vi "Host_continuousPathSamplingFPGA2.vi"() -> ()   [LabVIEW 2017]
uses:
  <vilib>/Utility/file.llb/Read From Spreadsheet File (I64).vi
  <vilib>/FPGAPlugInAG/cRIO-9082/niLvFpga_Open_cRIO-9082.vi
  <vilib>/rvi/interface/common/dynamic/niFpgaDynamicAddResources.vi
  <vilib>/FPGAPlugInAG/Dynamic/niLvFpga_Reset_Dynamic.vi
  <vilib>/Utility/error.llb/Error Cluster From Error Code.vi
  <vilib>/rvi/errors/niLvFpgaAdjustHostInterfaceError.vi
  <vilib>/rvi/interface/common/niFpgaWaitOnOcc.vi
  <vilib>/FPGAPlugInAG/Dynamic/niLvFpga_Run_Dynamic.vi
  <vilib>/Utility/file.llb/Write To Spreadsheet File (DBL).vi
  <vilib>/rvi/interface/nirviOpenFPGA/nirviOpenFPGA.xnode
  FPGA Bitfiles/simpletest_FPGATarget_coutinuousPathSa_wEIBsGw6M4w.lvbitx
  coutinuousPathSamplingFPGA4.vi
  <vilib>/rvi/interface/nirviMethod/nirviMethod.xnode
  <vilib>/rvi/interface/nirviReadWriteControl/nirviReadWriteControl.xnode
  <vilib>/rvi/interface/Simulation/niFpgaSimulationCallBeginRW.vi
  <vilib>/FPGAPlugInAG/Dynamic/niLvFpga_ConfigureFifo_Dynamic.vi
  <vilib>/rvi/errors/niLvFpgaMergeErrorWithErrorCode.vi
  NiFpgaLv.dll
  <vilib>/FPGAPlugInAG/Dynamic/niLvFpga_WriteFifo_Dynamic.vi
  <vilib>/FPGAPlugInAG/Dynamic/niLvFpga_StartFifo_Dynamic.vi
  <vilib>/FPGAPlugInAG/Dynamic/niLvFpga_ReadFifo_Dynamic.vi
panel:
  out "z output":dbl=5.1361083984375
  out "y output":dbl=3.794647216796875
  out "x output":dbl=-1.222381591796875
  out "deflection":dbl=-0.001068115234375
  out "z":dbl=-4.291839599609375
  out "y":dbl=3.9134521484375
  out "x":dbl=1.858306884765625
  out "Elements Remaining":u32=68432
  out "FINISH_SIGNAL":bool
  in  "stop":bool
  in  "scanning path file path":path=path "C:/Users/AnderssonLab/Desktop/yufan/sample locations/finalSamplingSeqRFD_continuous256MuPath50_8FOR14_1D2_1400_16ptg_1.txt"
  out "Empty Elements Remaining":u32
  out "Actual Depth":u32=24188
  in  "Threshold":T1={"x threshold"=0.02301025390625, "y threshold"=0.02301025390625, "z threshold"=0.5, "deflection threshold"=0.019989013671875}
  in  "ImageToSample":T2={"image size_x"=256, "image size_y"=256, "sample start_x"=0.0, "sample start_y"=0.0, "sample end_x"=6.0, "sample end_y"=6.0}
  in  "deflection control":T3={"SetPoint (V)"=0.0, "scanning I"=20.0, "scanning P"=0.01953125, "Initial I (V)"=0.0, "Upper Limit (V)"=9.900000095367432, "Lower Limit (V)"=-9.900000095367432}
  in  "z control":T4={"SetPoint (V)"=-1.0, "I"=100.0, "P"=0.0595703125, "Initial I (V)"=0.0, "Upper Limit (V)"=9.900000095367432, "Lower Limit (V)"=-9.900000095367432}
  in  "y control":T3={"SetPoint (V)"=0.0, "scanning I"=1850.0, "scanning P"=0.099609375, "Initial I (V)"=0.0, "Upper Limit (V)"=9.900000095367432, "Lower Limit (V)"=-9.900000095367432}
  in  "x control":T3={"SetPoint (V)"=0.0, "scanning I"=1850.0, "scanning P"=0.099609375, "Initial I (V)"=0.0, "Upper Limit (V)"=9.900000095367432, "Lower Limit (V)"=-9.900000095367432}
  in  "Clock (uSec)":T5={"XY Clock (uSec)"=20.0, "Z Clock (uSec)"=3.0, "Stage Clock (uSec)"=500.0, "muPathUpdate Clock (uSec)"=200.0, "Sampling Clock (uSec)"=4500.0, "pixel segment"=100}
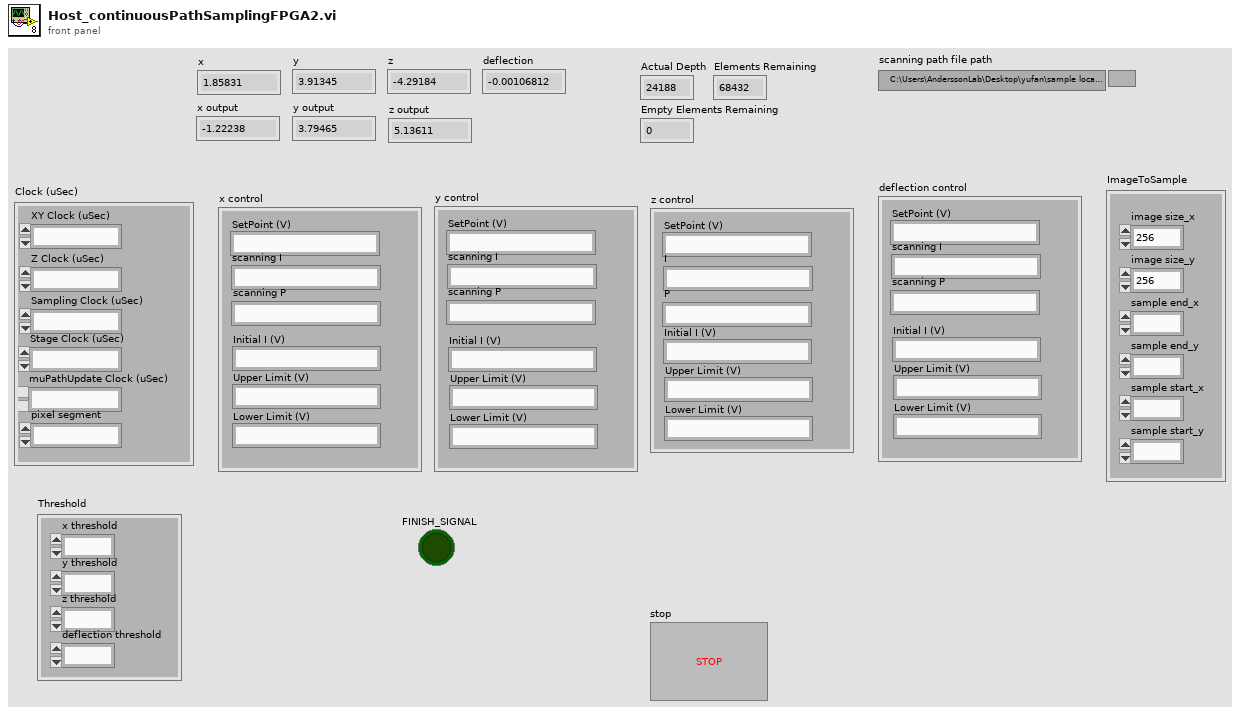
[diagram p1: front panel]
types:
  T1 = cluster{"x threshold":fxp<+/-,20,5>, "y threshold":fxp<+/-,20,5>, "z threshold":fxp<+/-,20,5>, "deflection threshold":fxp<+/-,20,5>}
  T2 = cluster{"image size_x":u16, "image size_y":u16, "sample start_x":fxp<+/-,26,5>, "sample start_y":fxp<+/-,26,5>, "sample end_x":fxp<+/-,26,5>, "sample end_y":fxp<+/-,26,5>}
  T3 = cluster{"SetPoint (V)":fxp<+/-,26,5>, "scanning I":fxp<+,21,13>, "scanning P":fxp<+,15,5>, "Initial I (V)":fxp<+/-,10,5>, "Upper Limit (V)":fxp<+/-,26,5>, "Lower Limit (V)":fxp<+/-,26,5>}
  T4 = cluster{"SetPoint (V)":fxp<+/-,26,5>, "I":fxp<+,21,13>, "P":fxp<+,15,5>, "Initial I (V)":fxp<+/-,10,5>, "Upper Limit (V)":fxp<+/-,26,5>, "Lower Limit (V)":fxp<+/-,26,5>}
  T5 = cluster{"XY Clock (uSec)":fxp<+,32,32>, "Z Clock (uSec)":fxp<+,32,32>, "Stage Clock (uSec)":fxp<+,32,32>, "muPathUpdate Clock (uSec)":fxp<+,32,32>, "Sampling Clock (uSec)":fxp<+,32,32>, "pixel segment":u32}
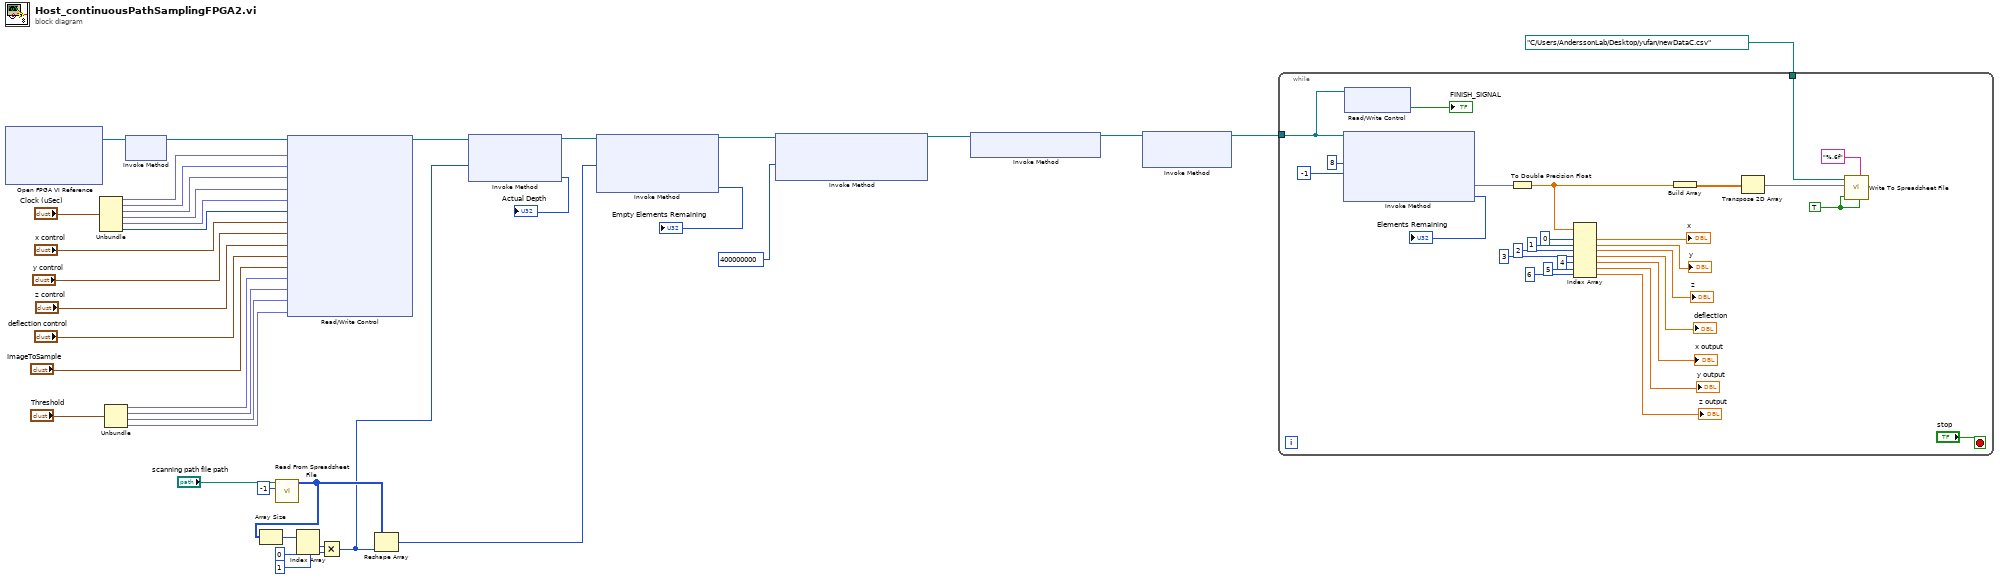
[diagram p0: block diagram]
diagram:
  n1 = xnode "Open FPGA VI Reference"() -> ("FPGA VI Reference Out"=w39:refnum<k20>)  [unwired: 2 in, 1 out]
  n2 = Unbundle("Clock (uSec)") -> ("XY Clock (uSec)"=w36:fxp<+,32,32>, "Z Clock (uSec)"=w35:fxp<+,32,32>, "Stage Clock (uSec)"=w34:fxp<+,32,32>, "muPathUpdate Clock (uSec)"=w33:fxp<+,32,32>, "Sampling Clock (uSec)"=w32:fxp<+,32,32>, "pixel segment"=w31:u32)
  n3 = Unbundle("Threshold") -> ("x threshold"=w24:fxp<+/-,20,5>, "y threshold"=w23:fxp<+/-,20,5>, "z threshold"=w22:fxp<+/-,20,5>, "deflection threshold"=w21:fxp<+/-,20,5>)
  n4 = xnode "Invoke Method"("FPGA VI Reference In"=w39) -> ("FPGA VI Reference Out"=w38:refnum<k20>)  [unwired: 1 in, 1 out]
  n5 = call-poly <vilib>:"Read From Spreadsheet File.vi"("number of rows (all:-1)"=-1, "file path (dialog if empty)"="scanning path file path") -> ("all rows"=w16:i64[][])  [unwired: 5 in, 4 out]
  n6 = Array Size(array=w16) -> (size(s)=w13:i32[])
  n7 = xnode "Read/Write Control"("FPGA VI Reference In"=w38, "XY Clock (uSec)"=w36, "Z Clock (uSec)"=w35, "Stage Clock (uSec)"=w34, "muPathUpdate Clock (uSec)"=w33, "Sampling Clock (uSec)"=w32, "pixel segment"=w31, "x control"="x control", "y control"="y control", "z control"="z control", "deflection control"="deflection control", "ImageToSample"="ImageToSample", "x threshold"=w24, "y threshold"=w23, "z threshold"=w22, "deflection threshold"=w21) -> ("FPGA VI Reference Out"=w20:refnum<k20>)  [unwired: 1 in, 1 out]
  n8 = Index Array(array=w13, index #1=0 ("index"), index #2=1 ("index")) -> (element #1=w14:i32, element #2=w15:i32)
  n9 = Multiply(x=w14, y=w15) -> (x*y=w8:i32)
  n10 = Reshape Array(w16, w8) -> (w7:i64[])
  n11 = xnode "Invoke Method"("FPGA VI Reference In"=w20, "Requested Depth"=w8) -> ("FPGA VI Reference Out"=w19:refnum<k20>, "Actual Depth"=→"Actual Depth":u32)  [unwired: 1 in, 1 out]
  n12 = xnode "Invoke Method"("FPGA VI Reference In"=w19, "Data"=w7) -> ("FPGA VI Reference Out"=w6:refnum<k20>, "Empty Elements Remaining"=→"Empty Elements Remaining":u32)  [unwired: 2 in, 1 out]
  n13 = xnode "Invoke Method"("FPGA VI Reference In"=w6, "Requested Depth"=u32 400000000) -> ("FPGA VI Reference Out"=w4:refnum<k20>)  [unwired: 1 in, 2 out]
  n14 = xnode "Invoke Method"("FPGA VI Reference In"=w4) -> ("FPGA VI Reference Out"=w3:refnum<k20>)  [unwired: 1 in, 1 out]
  n15 = xnode "Invoke Method"("FPGA VI Reference In"=w3) -> ("FPGA VI Reference Out"=w2:refnum<k20>)  [unwired: 2 in, 1 out]
  n16 = while {
    tunnel: w2 -> [w65]
    tunnel: path "C:/Users/AnderssonLab/Desktop/yufan/newDataC.csv" ("file path (dialog if empty)") -> [w40]
    stop <- "stop" stop-if-true
    w45 = TRUE
    n17 = xnode "Invoke Method"("FPGA VI Reference In"=w65, "Number of Elements"=u32 8, "Timeout (ms)"=-1) -> ("Data"=w53:fxp<+/-,25,5>[], "Elements Remaining"=→"Elements Remaining":u32)  [unwired: 1 in, 2 out]
    n18 = xnode "Read/Write Control"("FPGA VI Reference In"=w65) -> ("signalToStop"=→"FINISH_SIGNAL":bool)  [unwired: 1 in, 2 out]
    n19 = To Double Precision Float(number=w53) -> (double precision float=w41:dbl[])
    n20 = Index Array(array=w41, index #1=0 ("index"), index #2=1 ("index"), index #3=2 ("index"), index #4=3 ("index"), index #5=4 ("index"), index #6=5 ("index"), index #7=6 ("index")) -> (element #1=→"x":dbl, element #2=→"y":dbl, element #3=→"z":dbl, element #4=→"deflection":dbl, element #5=→"x output":dbl, element #6=→"y output":dbl, element #7=→"z output":dbl)
    n21 = Build Array(w41) -> (w43:dbl[][])
    n22 = Transpose 2D Array(2D array=w43) -> (transposed array=w42:dbl[][])
    n23 = call-poly <vilib>:"Write To Spreadsheet File.vi"("transpose? (no:F)"=w45, "format (%.3f)"="%.6f", "append to file? (new file:F)"=w45, "2D data"=w42, "file path (dialog if empty)"=w40) -> ()  [unwired: 3 in, 1 out]
  }
